vi "FileName.StripName.vi"(11 "filenames":string[](array[string])) -> (3 "File name (no extension)":string[](array[string]))   [LabVIEW 2015, in "Simple Sequence Tools - Shared.lvlib"]
uses:
  Simple Sequence Tools - Shared.lvlib
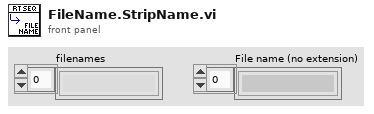
[diagram p1: front panel]
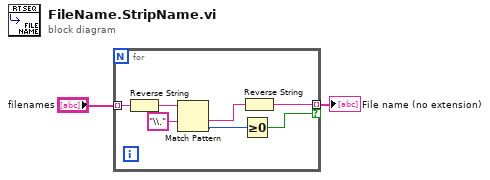
[diagram p0: block diagram]
diagram:
  n1 = for {
    tunnel: "filenames" -> [w7] mode=indexing
    tunnel: [w6] -> w2 mode=indexing if=w3
    n2 = Reverse String(1:w7) -> (0:w9:string)
    n3 = Match Pattern(string=w9, regular expression="\\.") -> (after substring=w5:string, offset past match=w4:i32)  [unwired: 1 in, 2 out]
    n4 = Greater Or Equal To 0?(x=w4) -> (x >= 0?=w3:bool)
    n5 = Reverse String(1:w5) -> (0:w6:string)
  }
  "File name (no extension)" <- w2
